vi "Dashboard Main.vi"() -> ()   [LabVIEW 2020]
uses:
  52f2dcef-b32f-41dc-9262-467f65fbdc6c.vi
  <vilib>/Rock Robotics/Network Tables/NT Write String Array.vi
  <vilib>/Rock Robotics/Network Tables/NT Write Boolean.vi
  <vilib>/Rock Robotics/WPI/Dashboard/WPI_DashboardLogging Global.vi
panel:
  out "NT Connection":bool
  in  "Camera Settings Right":T1={"Frame Rate"=30, "Compression"=30, "Size"=1, "DB Camera Config"=FALSE} {"Frame Rate" scale=1.0..30.0; "Compression" scale=100.0..-1.0; "Size" items=["640x480", "320x240", "160x120"]}
  in  "Camera Name Right":string(combo)="No Camera Selection"
  out "Camera Perf":string
  in  "TCP":refnum<k5>
  in  "Rec Mode":enum32{"Stop", "Record", "Playback"}(radio)
  out "Robot IP":string
  out "Image Message":string="Timeout in Camera Communications"
  in  "Dashboard Tab":T2(tab)
  in  "Balance in Manual?":bool=TRUE
  in  "Preload Cone?":bool=TRUE
  out "IMU Roll":dbl
  out "IMU Pitch":dbl
  in  "AE Speed":dbl=0.08
  in  "Config AE":bool=TRUE
  in  "Reset Wrist":bool
  in  "Reset Cascade":bool
  out "Wrist":dbl=15.0
  out "Cascade":dbl=0.1
  in  "Auto Calibrate":bool=TRUE
  in  "Robot Selector":u16(ring) items=["2468", "2687"]
  in  "Manual Paths":string[](array[string])
  in  "Max Rotation":dbl=270.0
  in  "Max Translation":dbl=16.0
  in  "Deadband":dbl=0.1
  in  "Auto Selector":T3(ring)
  out "IMU":dbl(knob) scale=-180.0..180.0
  in  "Select Auto":string(combo)="Select Autonomous ..."
  out "Mode":T4(ring)=enum."Auto Disabled"
  out "Right Camera Perf":cluster{"Bandwidth (Mbps)":dbl, "FPS":dbl}
  out "Auto Picture":picture
  out "Cone":bool
  out "Cube":bool
  in  "Mid":bool=TRUE
  in  "High":bool=TRUE
  in  "Field Centric":bool
  out "Camera Image Right":T5(plugin-control)
  out "Tree":string(tree)
  # "HW"
  # "IMU"
  # "SWERVE"
  # "PATH VISUAL"
  # "MANIPULATOR"
  # "CONFIGURATION"
  # "FIELD CENTRIC"
  # "HIGH"
  # "MID"
  # "CUBE"
  # "CONE"
  # "BRUSHLESS"
  # "12V MISSING"
  # "SENSOR FAULT"
  # "BRAKE"
  # "COAST"
  # "CAN FAULT"
  # "REVERSE"
  # "FORWARD"
  # "CORRUPT"
  # "UPDATING"
  # "RECOVERY"
  # "BRUSHED"
  # "BRAKE"
  # "COAST"
  # "https://cdn8.bigcommerce.com/s-t3eo8vwp22/product_images/uploaded_images/fault-no-12v.gif"
  # "PIGEON 2"
  # "DAMAGED HARDWARE"
  # "BOOTLOADER"
  # "CAN FAULT"
  # "ROBOT DISABLED"
  # "ROBOT ENABLED"
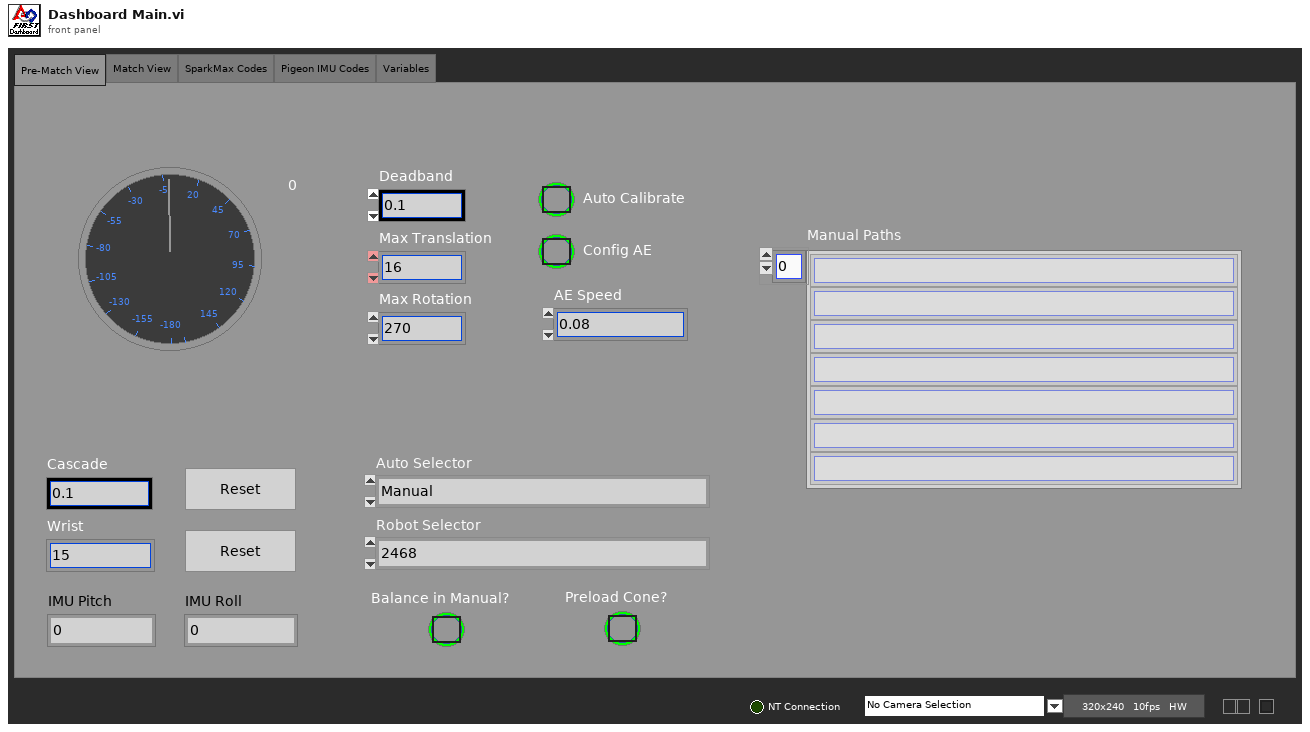
[diagram p1: front panel]
types:
  T1 = cluster{"Frame Rate":i32, "Compression":i32, "Size":u16, "DB Camera Config":bool}
  T2 = enum32{"Pre-Match View", "Match View", "SparkMax Codes", "Pigeon IMU Codes", "Variables"}
  T3 = enum16{"Manual", "FEEDER - 2.5 (2 High) + Balance", "FEEDER - 3 (2 High, 1 Low)", "WALL - 2 (High) + Balance", "WALL - 3 (2 High, 1 Low)", "MIDDLE - Wall Side 2 (High) + Balance", "MIDDLE - Feeder Side 2 (High) + Balance"}
  T4 = enum8{"Tele-Op Disabled", "Tele-Op Enabled", "Auto Disabled", "Auto Enabled", "Test Disabled", "Test Enabled", "Disconnected", "No Code", "E-Stop"}
  T5 = typedef "IMAQ Image.ctl" = refnum<image>
  T6 = cluster{"Save Path":path, "Interval (s)":dbl, "Keep":i32}
  T7 = typedef "Image Type" = u32
  T8 = cluster{"IDs":cluster{"RPC field ID":u16, "Unique ID":u16}, "String":string}
  T9 = cluster{"Dashboard Tab":refnum<vi>, "Rec Mode":refnum<vi>, "Tree":refnum<vi>, "Camera Perf":refnum<vi>, "Camera Settings Right":refnum<vi>, "Camera Name Right":refnum<vi>, "Camera Image Right":refnum<vi>}
  T10 = cluster{"Global Rectangle":i32[], "Contours":cluster{"Contour Type":u32, "ROI Type":u32, "Points":i32[]}[]}
  T11 = cluster{"Camera Name Right":string, string, "Saved DB Images Info":cluster{"Save Path":path, "Interval (s)":dbl, "Keep":i32}}
  T12 = cluster{"Error Strings":string, "Disable Counts":cluster{u16, u16}, "Rail Faults":cluster{u16, u16, u16}, "Robot IP":string, "DB Mode":u8, "Event Info":cluster{"Name":string, "Type":u8, "Number":u16, "Replay":u8}}
  T13 = cluster{"Storage":cluster{"Disk Free":u64, "RAM Block":u32, "RAM free":u32}, "CPU Utilization":cluster{"CPU % ISR":sgl, "CPU % Time Crit":sgl, "CPU % Timed Str":sgl, "CPU % High":sgl, "CPU % Above":sgl, "CPU % Normal":sgl, "CPU % Low":sgl}, "CAN":cluster{"% Bus Utilization":sgl, "Bus Off Cnt":u32, "TX_FIFO Full Cnt":u32, "Receive Error Cnt":u8, "Transmit Error Cnt":u8}, "HID":cluster{"HID Outputs":u32, "Rumble Low":u16, "Rumble High":u16}[]}
  T14 = cluster{"Status bits":cluster{"Test Mode":bool, "Autonomous":bool, "Enabled":bool, "Code Start":bool, "Brownout":bool, "Reserved 2":bool, "Reserved 3":bool, "E-Stop":bool}, "Code Trace":cluster{"Disabled":bool, "TeleOp":bool, "Auto":bool, "Test":bool}, "Controller Type":enum16{"unknown", "cRIO", "roboRio"}, "Code?":enum16{"unknown", "noCode", "code"}, "Battery V":dbl}
  T15 = cluster{"Control Bits":cluster{"TestMode":bool, "Autonomous":bool, "Enabled":bool, "FMS Present":bool, bool, bool, bool, "E-Stop":bool}, "Team Station ":u8, "Countdown":sgl, "Joystick Values":cluster{"Axes":dbl[], "Buttons":bool[], "POVs":i16[]}[]}
  T16 = typedef "imagedata.ctl" = cluster{"image type":i32, "image depth":i32, "image":u8[], "mask":u8[], "colors":u32[], "Rectangle":cluster{"left":i16, "top":i16, "right":i16, "bottom":i16}}
  T17 = cluster{"Operation":enum16{"Update", "Clear"}, "Color Box":u32}[]
  T18 = cluster{"Image Size":bool, "Image Type":bool, "Pixel Value":bool, "ROI Information":bool, "Zoom Factor":bool}
  T19 = cluster{"Shift":bool, "Ctrl":bool, "Alt":bool, "Cmd":bool, "Opt":bool}
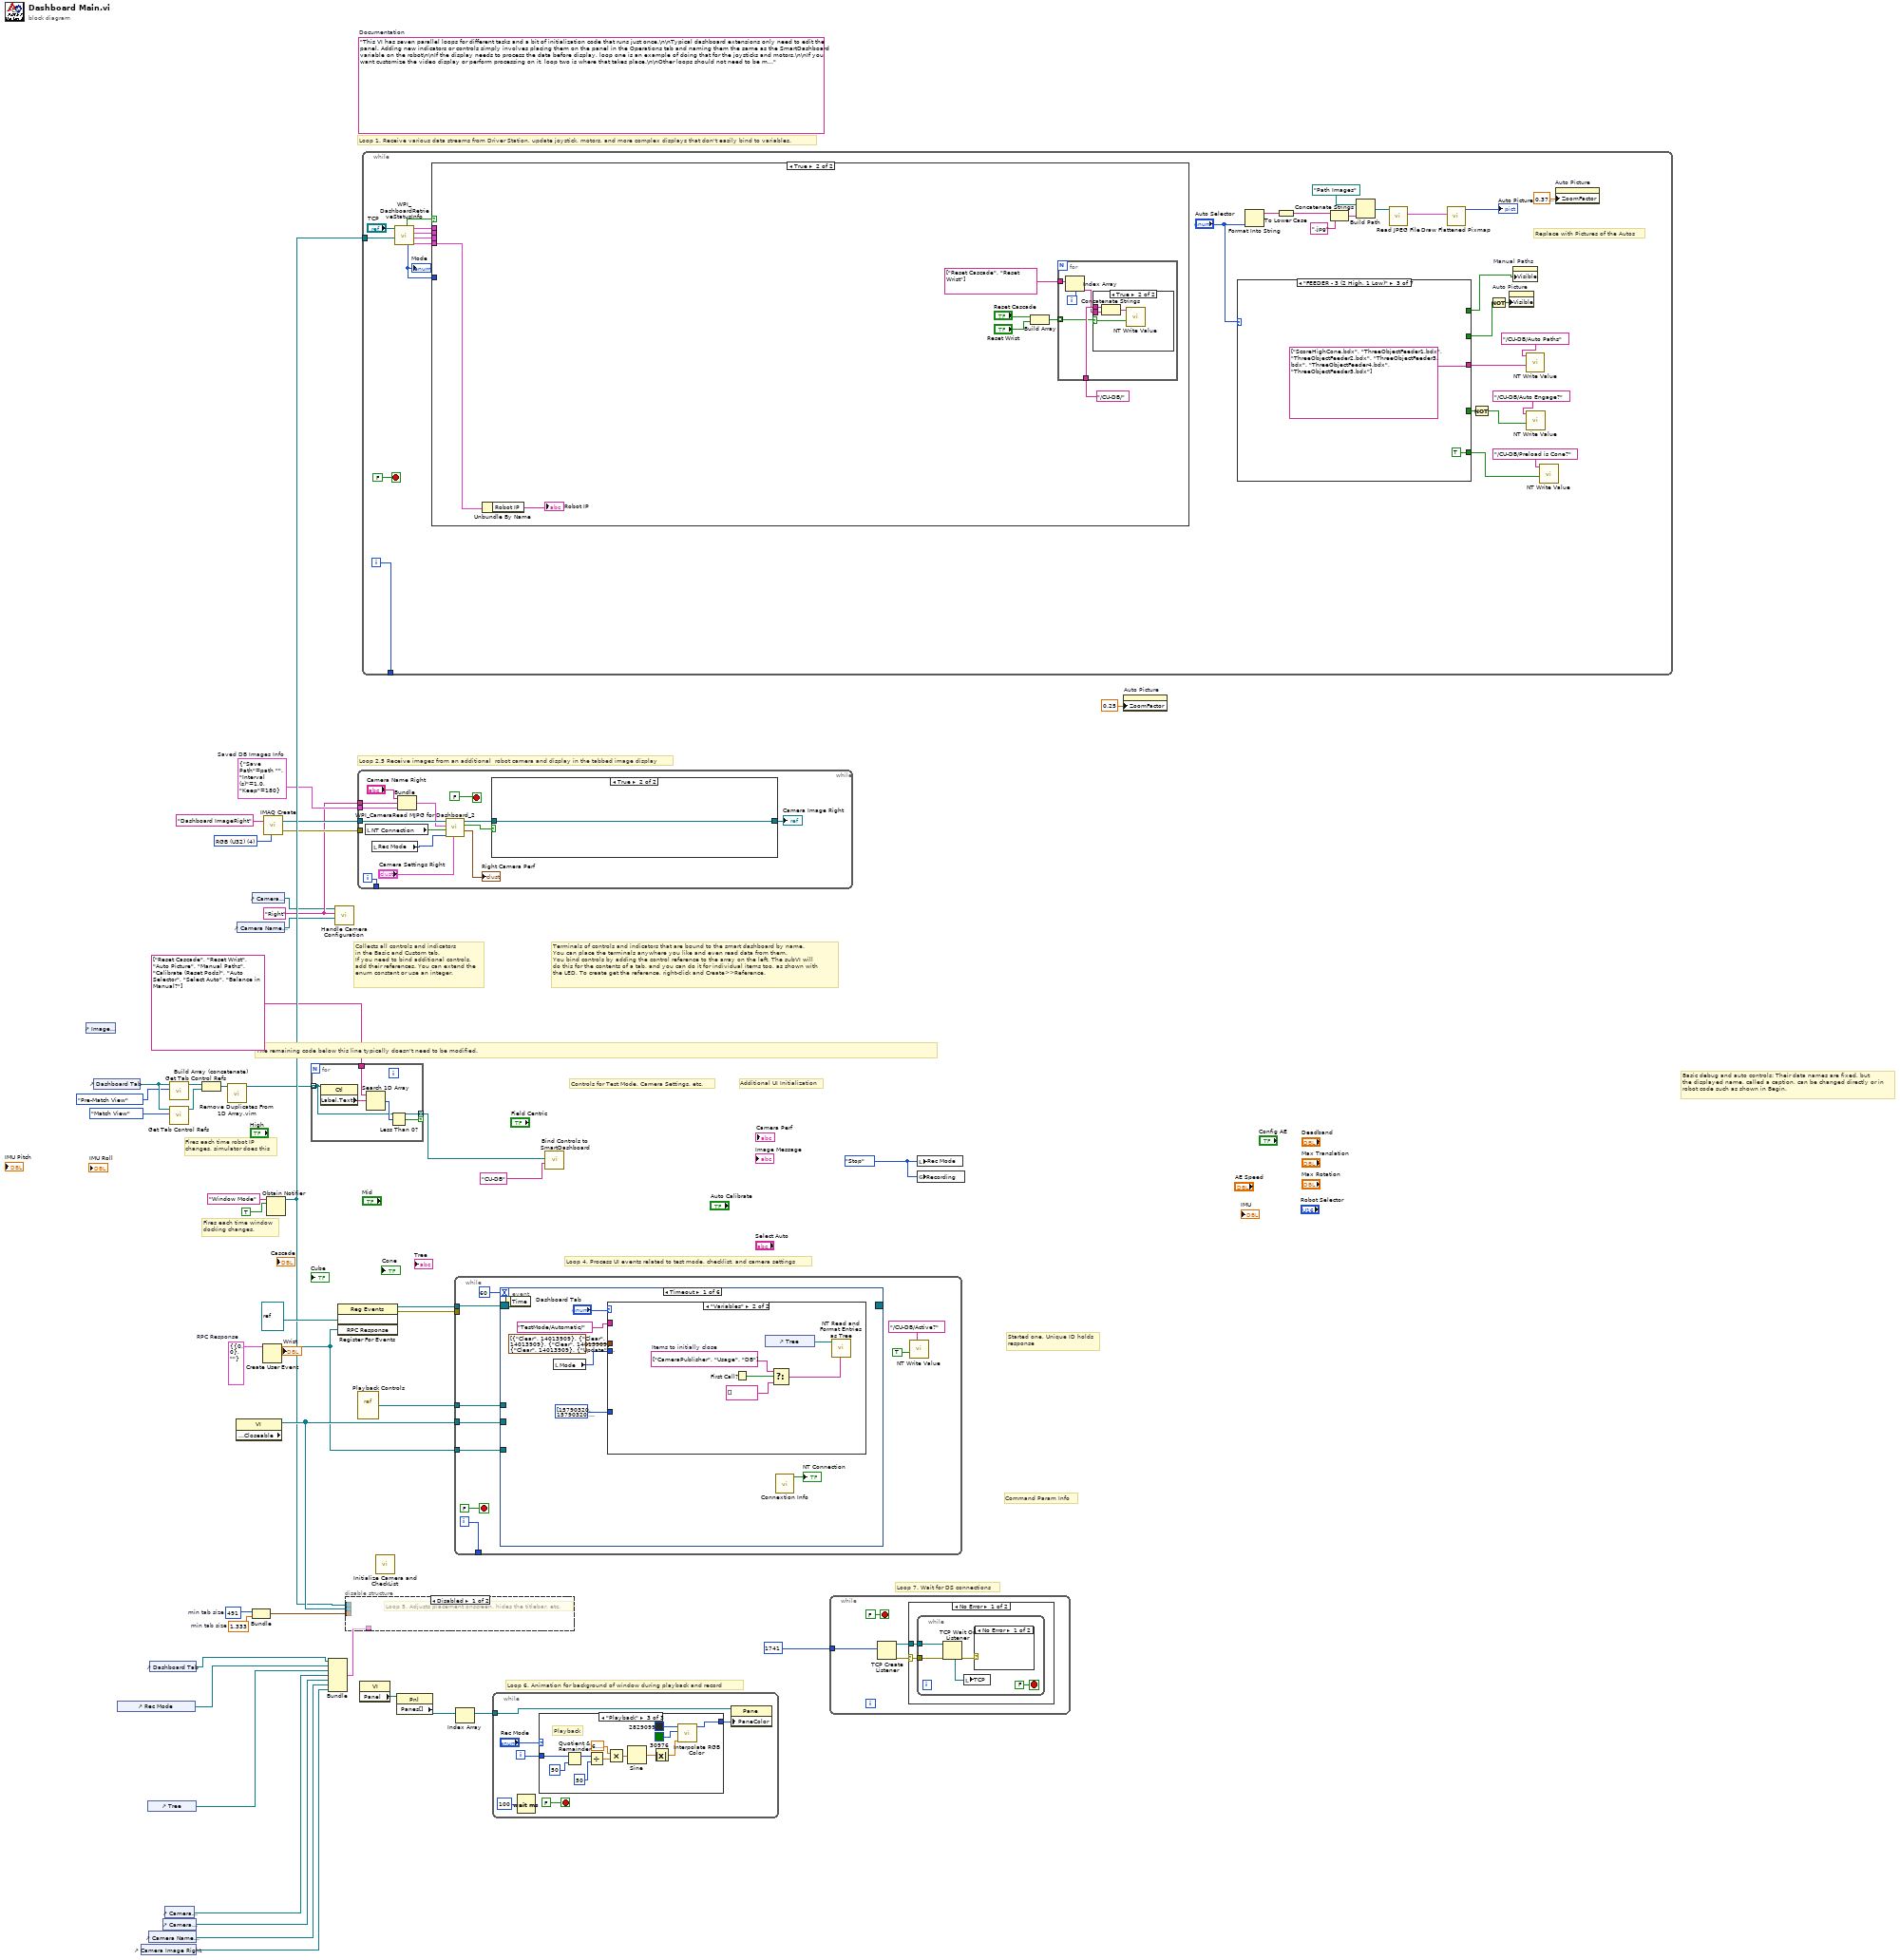
[diagram p0: block diagram]
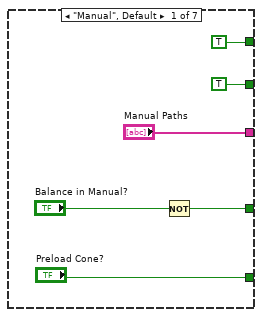
[diagram p2: hidden frame]
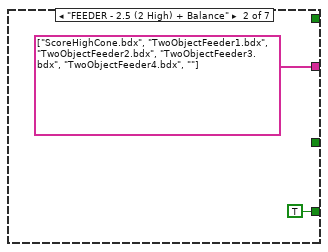
[diagram p3: hidden frame]
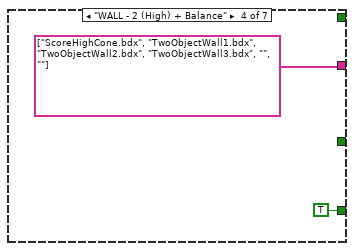
[diagram p4: hidden frame]
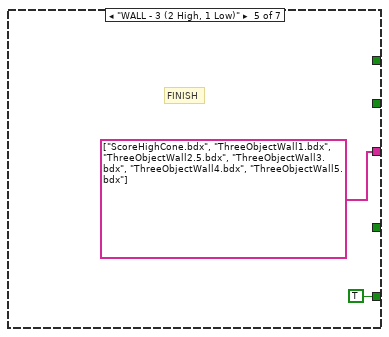
[diagram p5: hidden frame]
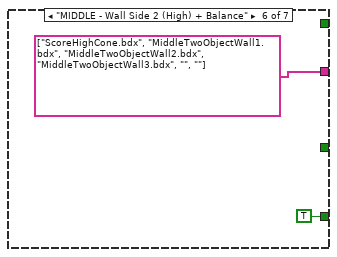
[diagram p6: hidden frame]
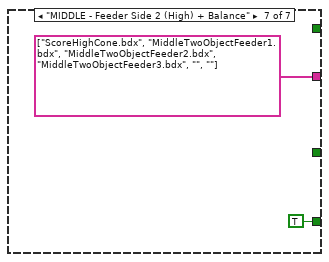
[diagram p7: hidden frame]
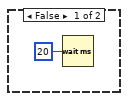
[diagram p8: hidden frame]
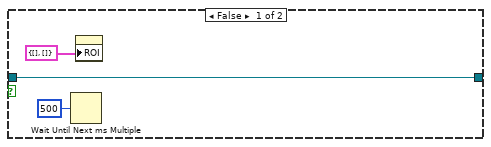
[diagram p11: hidden frame]
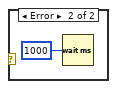
[diagram p12: hidden frame]
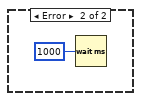
[diagram p13: hidden frame]
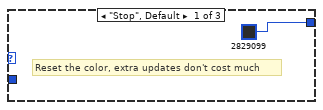
[diagram p14: hidden frame]
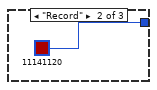
[diagram p15: hidden frame]
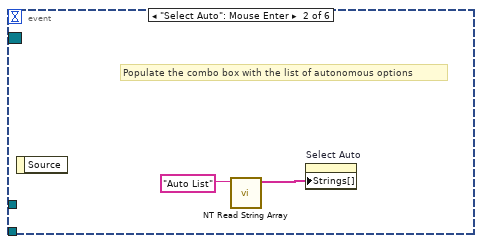
[diagram p17: hidden frame]
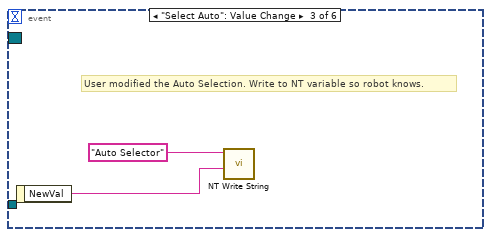
[diagram p18: hidden frame]
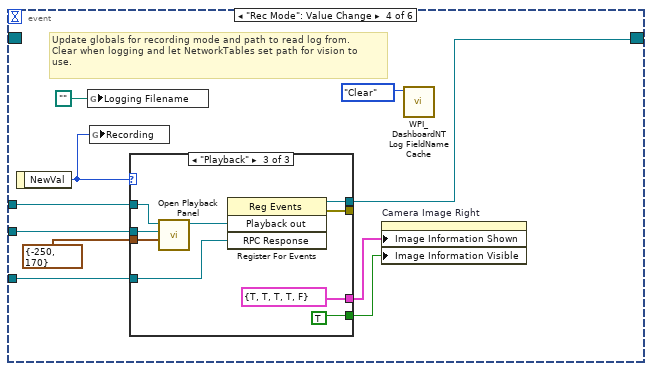
[diagram p19: hidden frame]
diagram:
  w17 = T6 {"Save Path"=path "", "Interval (s)"=1.0, "Keep"=180}  # Saved DB Images Info
  w16 = "Right"
  w23 = T7 4 items=["Grayscale (U8)", "Grayscale (I16)", "Grayscale (SGL)", "Complex (CSG)", "RGB (U32)", "HSL (U32)", "RGB (U64)"] ("Image Type")
  w27 = T8 {"IDs"={"RPC field ID"=0, "Unique ID"=0}, "String"=""}  # RPC Response
  w34 = 491  # min tab size
  w33 = 1.333  # min tab size
  w36 = enum32{"Stop", "Record", "Playback"}."Stop" ("Rec Mode")
  (unwired) "This VI has seven parallel loops for different tasks and a bit of initialization code that runs just once.\n\nTypical dashboard extensions only need to edit the panel. Adding new indicators or controls simply involves placing them on the panel in the Operations tab and naming them the same as the SmartDashboard variable on the robot\n\nIf the display needs to process the data before display, loop one is an example of doing that for the joysticks and motors.\n\nIf you want customize the video display or perform processing on it, loop two is where that takes place.\n\nOther loops should not need to be modified. They are pretty standard, and document the task they perform."  # Documentation
  # "Loop 2.5 Receive images from an additional  robot camera and display in the tabbed image display"
  # "Command Param Info"
  # "Started one, Unique ID holds\nresponse"
  # "Loop 7. Wait for DS connections"
  # "Basic debug and auto controls: Their data names are fixed, but\nthe displayed name, called a caption, can be changed directly or in\nrobot code such as shown in Begin."
  # "Controls for Test Mode, Camera Settings, etc."
  # "Additional UI Initialization"
  # "Loop 6. Animation for background of window during playback and record"
  # "Fires each time robot IP\nchanges, simulator does this"
  # "Fires each time window\ndocking changes."
  # "Collects all controls and indicators\nin the Basic and Custom tab.\nIf you need to bind additional controls,\nadd their references. You can extend the\nenum constant or use an integer."
  # "The remaining code below this line typically doesn't need to be modified."
  # "Loop 4. Process UI events related to test mode, checklist, and camera settings"
  # "Terminals of controls and indicators that are bound to the smart dashboard by name.\nYou can place the terminals anywhere you like and even read data from them.\nYou bind controls by adding the control reference to the array on the left. The subVI will\ndo this for the contents of a tab, and you can do it for individual items too, as shown with\nthe LED. To create get the reference, right-click and Create>>Reference."
  # "Loop 1. Receive various data streams from Driver Station, update joystick, motors, and more complex displays that don't easily bind to variables."
  n1 = control-ref of="Image Message"() -> ()  [unwired: 1 out]
  n2 = control-ref of="Dashboard Tab"() -> (w13:refnum<vi>)
  n3 = control-ref of="Rec Mode"() -> (w30:refnum<vi>)
  n4 = control-ref of="Camera Image Right"() -> (w18:refnum<vi>)
  n5 = control-ref of="Tree"() -> (w15:refnum<vi>)
  n6 = control-ref of="Camera Name Right"() -> (w19:refnum<vi>)
  n7 = control-ref of="Dashboard Tab"() -> (w5:refnum<vi>)
  n8 = control-ref of="Camera Settings Right"() -> (w20:refnum<vi>)
  n9 = control-ref of="Camera Perf"() -> (w25:refnum<vi>)
  n10 = call <vilib>:"Get Tab Control Refs.vi"("Page Index"=T2."Pre-Match View" ("Dashboard Tab"), "TabControl in"=w13) -> ("ControlsOnPage"=w12:refnum<vi>[])  [unwired: 9 in]
  n11 = call <vilib>:"Get Tab Control Refs.vi"("Page Index"=T2."Match View" ("Dashboard Tab"), "TabControl in"=w13) -> ("ControlsOnPage"=w11:refnum<vi>[])  [unwired: 9 in]
  n12 = Build Array (concatenate)(w12, w11) -> (w10:refnum<vi>[])
  n13 = call "Remove Duplicates From 1D Array.vim"("array"=w10) -> ("array with duplicates removed"=w7:refnum<vi>[])  [unwired: 10 in]
  n14 = property class="VI" props=["Front Panel.Closeable"]() -> (reference out=w35:refnum<vi>)  [unwired: 2 in, 2 out]
  n15 = control-ref of="Camera Name Right"() -> (w1:refnum<vi>)
  n16 = control-ref of="Camera Settings Right"() -> (w2:refnum<vi>)
  n17 = Bundle("min tab size"=w34, "min tab size"=w33) -> (w32:cluster{"min tab size":i32, "min tab size":dbl})  [unwired: 1 in]
  n18 = Create User Event(user event datatype=w27) -> (user event=w26:refnum<user-event>)  [unwired: 1 in, 1 out]
  n19 = call "IMAQ Create"("Image Name"="Dashboard ImageRight", "Image Type"=w23) -> ("New Image"=w22:T5, "error out"=w21:errorcluster)  [unwired: 2 in, 1 out]
  n20 = Obtain Notifier(name (unnamed)="Window Mode", notification data type=TRUE) -> (notifier out=w29:refnum<notifier>)  [unwired: 2 in, 2 out]
  n21 = for {
    tunnel: string[] ["Reset Cascade", "Reset Wrist", "Auto Picture", "Manual Paths", "Calibrate (Reset Pods)", "Auto Selector", "Select Auto", "Balance in Manual?"] -> [w50]
    tunnel: w7 -> [w47] mode=indexing
    tunnel: [w47] -> w6 mode=indexing if=w46
    n22 = property class="Ctl"(reference=w47) -> ("Label.Text"=w49:string)  [unwired: 1 in, 2 out]
    n23 = Search 1D Array(1D array=w50, element=w49) -> (index of element=w48:i32)  [unwired: 1 in]
    n24 = Less Than 0?(x=w48) -> (x < 0?=w46:bool)
  }
  n25 = Bundle("Dashboard Tab"=w5, "Rec Mode"=w30, "Tree"=w15, "Camera Perf"=w25, "Camera Settings Right"=w20, "Camera Name Right"=w19, "Camera Image Right"=w18) -> (w31:T9)  [unwired: 1 in]
  n26 = call "Handle Camera Configuration.vi"("CameraNameRef"=w1, "Display Name"=w16, "ClusterRef"=w2) -> ()  [unwired: 9 in]
  n27 = register-events(refnum<vi> refnum, w26) -> (reference out=w39:refnum<event-registration>, error out=w38:errorcluster)  [unwired: 2 in]
  n28 = disable-structure shown="Disabled" {
    disable-tunnel: w35 -> [_ _]
    disable-tunnel: w32 -> [_ _]
    disable-tunnel: w31 -> [_ _]
    disable-tunnel: w29 -> [_ _]
    frame Disabled {
      # "Loop 5. Adjusts placement onscreen, hides the titlebar, etc."
    }
    frame Enabled {
    }
  }
  n29 = while {
    tunnel: w22 -> [w64]
    tunnel: w21 -> [_]
    tunnel: [w59] -> _
    tunnel: w17 -> [w55]
    tunnel: w16 -> [w52]
    i -> [w59]
    stop <- FALSE stop-if-true
    n30 = local read "NT Connection"() -> (w56:bool)
    n31 = local read "Rec Mode"() -> (w63:enum32{"Stop", "Record", "Playback"})
    n32 = Bundle("Camera Name Right"="Camera Name Right", w52, "Saved DB Images Info"=w55) -> (w54:T11)  [unwired: 1 in]
    n33 = call <vilib>:"WPI_CameraRead MJPG for Dashboard_2.vi"("Camera Settings"="Camera Settings Right", "Rec Mode"=w63, "NT Connection"=w56, "Capture Info"=w54, "Image in"=w64) -> ("perf info"=→"Right Camera Perf":cluster{"Bandwidth (Mbps)":dbl, "fps":dbl}, "Active"=w58:bool, "Image\\ out"=w61:T5)  [unwired: 4 in]
    n34 = case shown="True" w58 {
      tunnel: w61 -> [w66 w68]
      tunnel: [w66 w68] -> w57
      frame False {
        n35 = Wait Until Next ms Multiple(millisecond multiple=u32 500) -> ()  [unwired: 1 out]
        n36 = property on="Camera Image Right" class="ImageControl"("ROI"=T10 {"Global Rectangle"=[], "Contours"=[]}) -> ()  [unwired: 2 in, 2 out]
      }
      frame True {
      }
    }
    "Camera Image Right" <- w57
  }
  n37 = vi-ref "Playback Controls.vi"() -> (w40:refnum<vi>)
  n38 = property class="VI"() -> ("Panel"=w42:refnum<vi>)  [unwired: 2 in, 2 out]
  n39 = while {
    tunnel: [w97] -> _
    tunnel: w29 -> [w89]
    i -> [w97]
    stop <- FALSE stop-if-true
    # "Replace with Pictures of the Autos"
    n40 = call <vilib>:"WPI_DashboardRetrieveStatusInfo.vi"("Window Mode Notifier"=w89, "TCP Cnx"="TCP") -> ("Power and Errors"=w92:T12, "Robot Metrics"=w95:T13, "Status Info"=w96:T14, "Control Info"=w93:T15, "Robot Mode"=w91:T4, "Process?"=w94:bool)  [unwired: 4 in]
    "Mode" <- w91
    n41 = case shown="True" w94 {
      tunnel: w96 -> [_ _]
      tunnel: w95 -> [_ _]
      tunnel: w93 -> [_ _]
      tunnel: w92 -> [_ w124]
      tunnel: w91 -> [_ _]
      frame False {
        n42 = Wait (ms)(milliseconds to wait=u32 20) -> ()  [unwired: 1 out]
      }
      frame True {
        n43 = Unbundle By Name(w124) -> ("Robot IP"=→"Robot IP":string)
        n44 = Build Array("Reset Cascade", "Reset Wrist") -> (w118:bool[])
        n45 = for {
          tunnel: "/CU-DB/" ("Name") -> [w129]
          tunnel: w118 -> [w125] mode=indexing
          tunnel: string[] ["Reset Cascade", "Reset Wrist"] -> [w127]
          i -> [w128]
          n46 = Index Array(array=w127, index=w128) -> (element=w126:string)
          n47 = case shown="True" w125 {
            selector: w125 -> [_ w130]
            tunnel: w129 -> [_ w132]
            tunnel: w126 -> [_ w131]
            frame False {
            }
            frame True {
              n48 = Concatenate Strings(w132, w131) -> (w133:string)
              n49 = call-poly <vilib>:"NT Write Value.vi"("value"=w130, "name"=w133) -> ()  [unwired: 9 in, 1 out]
            }
          }
        }
      }
    }
    n50 = case shown="\"FEEDER - 3 (2 High, 1 Low)\"" "Auto Selector" {
      tunnel: ["Manual Paths" string[] ["ScoreHighCone.bdx", "TwoObjectFeeder1.bdx", "TwoObjectFeeder2.bdx", "TwoObjectFeeder3.bdx", "TwoObjectFeeder4.bdx", ""] ("Manual Paths") string[] ["ScoreHighCone.bdx", "ThreeObjectFeeder1.bdx", "ThreeObjectFeeder2.bdx", "ThreeObjectFeeder3.bdx", "ThreeObjectFeeder4.bdx", "ThreeObjectFeeder5.bdx"] ("Manual Paths") string[] ["ScoreHighCone.bdx", "TwoObjectWall1.bdx", "TwoObjectWall2.bdx", "TwoObjectWall3.bdx", "", ""] ("Manual Paths") string[] ["ScoreHighCone.bdx", "ThreeObjectWall1.bdx", "ThreeObjectWall2.5.bdx", "ThreeObjectWall3.bdx", "ThreeObjectWall4.bdx", "ThreeObjectWall5.bdx"] ("Manual Paths") string[] ["ScoreHighCone.bdx", "MiddleTwoObjectWall1.bdx", "MiddleTwoObjectWall2.bdx", "MiddleTwoObjectWall3.bdx", "", ""] ("Manual Paths") string[] ["ScoreHighCone.bdx", "MiddleTwoObjectFeeder1.bdx", "MiddleTwoObjectFeeder2.bdx", "MiddleTwoObjectFeeder3.bdx", "", ""] ("Manual Paths")] -> w83
      tunnel: [TRUE ("Visible") _ _ _ _ _ _] -> w82
      tunnel: [TRUE ("Visible") _ _ _ _ _ _] -> w81
      tunnel: [w101 _ _ _ _ _ _] -> w86
      tunnel: ["Preload Cone?" TRUE ("Preload is Cone?") TRUE ("Preload is Cone?") TRUE ("Preload is Cone?") TRUE ("Preload is Cone?") TRUE ("Preload is Cone?") TRUE ("Preload is Cone?")] -> w88
      frame "Manual", Default {
        n51 = Not(x="Balance in Manual?") -> (.not. x?=w101:bool)
      }
      frame "FEEDER - 2.5 (2 High) + Balance" {
      }
      frame "FEEDER - 3 (2 High, 1 Low)" {
      }
      frame "WALL - 2 (High) + Balance" {
      }
      frame "WALL - 3 (2 High, 1 Low)" {
        # "FINISH"
      }
      frame "MIDDLE - Wall Side 2 (High) + Balance" {
      }
      frame "MIDDLE - Feeder Side 2 (High) + Balance" {
      }
    }
    n52 = Format Into String("Auto Selector") -> (resulting string=w75:string)  [unwired: 3 in, 1 out]
    n53 = To Lower Case(string=w75) -> (all lower case string=w76:string)
    n54 = Concatenate Strings(w76, ".jpg" ("string")) -> (w77:string)
    n55 = Build Path(base path=path "Path Images", name or relative path=w77) -> (appended path=w85:path)
    n56 = call <vilib>:"Read JPEG File.vi"("path to JPEG file"=w85) -> ("image data"=w84:T16)  [unwired: 8 in, 2 out]
    n57 = call <vilib>:"Draw Flattened Pixmap.vi"("image data"=w84) -> ("new picture"=→"Auto Picture":picture)  [unwired: 8 in]
    n58 = Not(x=w86) -> (.not. x?=w87:bool)
    n59 = Not(x=w82) -> (.not. x?=w79:bool)
    n60 = property on="Auto Picture" class="Pict"("Visible"=w79) -> ()  [unwired: 2 in, 2 out]
    n61 = property on="Manual Paths" class="Arr (strict)"("Visible"=w81) -> ()  [unwired: 2 in, 2 out]
    n62 = call-poly <vilib>:"NT Write Value.vi"("value"=w83, "name"="/CU-DB/Auto Paths") -> ()  [unwired: 9 in, 1 out]
    n63 = call-poly <vilib>:"NT Write Value.vi"("value"=w87, "name"="/CU-DB/Auto Engage?") -> ()  [unwired: 9 in, 1 out]
    n64 = call-poly <vilib>:"NT Write Value.vi"("value"=w88, "name"="/CU-DB/Preload is Cone?") -> ()  [unwired: 9 in, 1 out]
    n65 = property on="Auto Picture" class="Pict"("ZoomFactor"=sgl 0.38 ("Zoom Factor")) -> ()  [unwired: 2 in, 2 out]
  }
  n66 = call "Initialize Camera and CheckList.vi"() -> ()  [unwired: 12 in]
  n67 = property class="Pnl"(reference=w42) -> ("Panes[]"=w43:refnum<vi>[])  [unwired: 1 in, 2 out]
  n68 = while {
    tunnel: [w140] -> _
    tunnel: w40 -> [w139]
    tunnel: w39 -> [w138]
    tunnel: w38 -> [_]
    tunnel: w35 -> [w137]
    tunnel: w26 -> [w136]
    i -> [w140]
    stop <- FALSE stop-if-true
    n69 = event shown="[0] Timeout" {
      selector: w138 -> [_ _ _ _ _ _]
      dyn-events: [_ _ _ w164 _ _] -> _
      timeout: u32 60 ("milliseconds to wait") -> [_ _ _ _ _ _]
      tunnel: w139 -> [_ _ _ w166 w181 _]
      tunnel: w137 -> [_ _ _ w162 _ _]
      tunnel: w136 -> [_ _ _ w160 _ _]
      event Timeout {
        n70 = event-data() -> ()  [unwired: 1 in, 1 out]
        n71 = local read "Mode"() -> (w145:T4)
        n72 = case shown="\"Variables\"" "Dashboard Tab" {
          tunnel: "TestMode/Automatic/" ("Name Pattern") -> [_ _]
          tunnel: T17 [{"Operation"=enum."Clear", "Color Box"=14013909}, {"Operation"=enum."Clear", "Color Box"=14013909}, {"Operation"=enum."Clear", "Color Box"=14013909}, {"Operation"=enum."Clear", "Color Box"=14013909}, {"Operation"=enum."Update", "Color Box"=14013909}, {"Operation"=enum."Update", "Color Box"=16777215}, {"Operation"=enum."Clear", "Color Box"=14013909}, {"Operation"=enum."Clear", "Color Box"=14013909}, {"Operation"=enum."Clear", "Color Box"=14013909}] -> [_ _]
          tunnel: w145 -> [_ _]
          tunnel: u32[] [15790320, 15790320, 15790320, 15790320, 16777215, 16777215, 15790320, 15790320, 15790320] -> [_ _]
          frame Default {
          }
          frame "Variables" {
            w151 = string[] ["CameraPublisher", "Usage", "DB"]  # Items to initially close
            n73 = First Call?() -> (First Call?: T/F=w152:bool)
            n74 = control-ref of="Tree"() -> (w153:refnum<vi>)
            n75 = Select(t=w151, s=w152, f=string[] []) -> (s? t:f=w149:string[])
            n76 = call <vilib>:"NT Read and Format Entries as Tree.vi"("Tags to  Close"=w149, "Tree Refnum"=w153) -> ()  [unwired: 8 in, 2 out]
          }
        }
        n77 = call <vilib>:"Connextion Info.vi"() -> ("Connected"=→"NT Connection":bool)  [unwired: 10 in, 1 out]
      }
      event "Select Auto": Mouse Enter {
        # "Populate the combo box with the list of autonomous options"
        n78 = event-data() -> ()  [unwired: 1 in, 1 out]
        n79 = call <vilib>:"NT Read String Array.vi"("name"="Auto List" ("Name")) -> ("value"=w154:string[])  [unwired: 8 in, 2 out]
        n80 = property on="Select Auto" class="CmbBox"("Strings[]"=w154) -> ()  [unwired: 2 in, 2 out]
      }
      event "Select Auto": Value Change {
        # "User modified the Auto Selection. Write to NT variable so robot knows."
        n81 = event-data() -> ("NewVal"=w156:string)  [unwired: 1 in]
        n82 = call <vilib>:"NT Write String.vi"("value"=w156, "name"="Auto Selector" ("Name")) -> ()  [unwired: 9 in, 1 out]
      }
      event "Rec Mode": Value Change {
        # "Update globals for recording mode and path to read log from.\nClear when logging and let NetworkTables set path for vision to\nuse."
        n83 = event-data() -> ("NewVal"=w167:enum32{"Stop", "Record", "Playback"})  [unwired: 1 in]
        n84 = global write "WPI_DashboardLogging Global.vi" "Logging Filename"(path "") -> ()
        n85 = global write "WPI_DashboardLogging Global.vi" "Recording"(w167) -> ()
        n86 = case shown="\"Playback\"" w167 {
          tunnel: w166 -> [_ w169 w178]
          tunnel: [_ _ w177] -> w164
          tunnel: [_ _ w176] -> _
          tunnel: w162 -> [_ _ w174]
          tunnel: cluster{i32, i32} {-250, 170} -> [_ _ w173]
          tunnel: [_ _ T18 {"Image Size"=TRUE, "Image Type"=TRUE, "Pixel Value"=TRUE, "ROI Information"=TRUE, "Zoom Factor"=FALSE} ("Image Information Shown:All Elements")] -> w158
          tunnel: [_ _ TRUE ("Zoom Factor")] -> w159
          tunnel: w160 -> [_ _ w170]
          frame Default {
          }
          frame "Stop", "Record" {
            # "Place Window too"
            n87 = invoke class="VI" method="FP.Close"(reference=w169) -> (reference out=w168:refnum<vi>)  [unwired: 2 in, 2 out]
            n88 = invoke class="VI" method="Abort VI"(reference=w168) -> ()  [unwired: 2 in, 3 out]
          }
          frame "Playback" {
            n89 = call "Open Playback Panel.vi"("Offset"=w173, "DB VI Ref"=w174, "Playback in"=w178) -> ("Playback out"=w175:refnum<vi>)  [unwired: 8 in]
            n90 = register-events(w175, w170) -> (reference out=w177:refnum<event-registration>, error out=w176:errorcluster)  [unwired: 2 in]
          }
        }
        n91 = property on="Camera Image Right" class="ImageControl"("Image Information Shown"=w158, "Image Information Visible"=w159) -> ()  [unwired: 2 in, 2 out]
        n92 = call <vilib>:"WPI_DashboardNT Log FieldName Cache.vi"("Operation"=enum16{"Lookup/Add", "Index", "Clear"}."Clear") -> ()  [unwired: 8 in, 3 out]
      }
      event Panel Close {
        # "Abort playback window and ourself"
        n93 = event-data() -> ()  [unwired: 1 in, 4 out]
        n94 = invoke class="VI" method="FP.Close"(reference=w181) -> (reference out=w180:refnum<vi>)  [unwired: 2 in, 2 out]
        n95 = invoke class="VI" method="Abort VI"(reference=w180) -> (error out=w179:errorcluster)  [unwired: 2 in, 2 out]
        n96 = invoke class="VI" method="Abort VI"(error in=w179) -> ()  [unwired: 2 in, 3 out]
      }
      event "Tree": Double Click {
        n97 = event-data() -> ("PlatMods"=w187:T19, "Tag"=w184:string)  [unwired: 1 in]
        n98 = Unbundle(w187) -> ("Shift"=w186:bool)  [unwired: 4 out]
        n99 = String Subset(string=w184, length (rest)=1 ("length (rest)")) -> (substring=w183:string)  [unwired: 1 in]
        n100 = Not(x=w186) -> (.not. x?=w185:bool)
        n101 = case shown="\"/\"" w183 {
          tunnel: w184 -> [_ w189]
          tunnel: w185 -> [_ w188]
          frame Default {
          }
          frame "/" {
            n102 = call <vilib>:"NT Update Persistence.vi"("Persistence"=w188, "Name"=w189) -> ()  [unwired: 9 in, 1 out]
          }
        }
      }
    }
    n103 = call-poly <vilib>:"NT Write Value.vi"("value"=TRUE ("Boolean"), "name"="/CU-DB/Active?" ("Name")) -> ()  [unwired: 9 in, 1 out]
  }
  n104 = Index Array(array=w43) -> (element=w41:refnum<vi>)  [unwired: 1 in]
  n105 = while {
    tunnel: w41 -> [w191]
    i -> [w194]
    stop <- FALSE stop-if-true
    n106 = Wait (ms)(milliseconds to wait=u32 100) -> ()  [unwired: 1 out]
    n107 = case shown="\"Playback\"" "Rec Mode" {
      tunnel: w194 -> [_ _ w209]
      tunnel: [u32 2829099 ("Base Color") u32 11141120 ("Target Color") w198] -> w190
      frame "Stop", Default {
        # "Reset the color, extra updates don't cost much"
      }
      frame "Record" {
      }
      frame "Playback" {
        # "Playback"
        n108 = Quotient & Remainder(x=w209, y=u32 50 ("milliseconds to wait")) -> (x-y*floor(x/y)=w205:u32)  [unwired: 1 out]
        n109 = Divide(x=w205, y=u32 50 ("milliseconds to wait")) -> (x/y=w202:dbl)
        n110 = Multiply(x=6.283185307179586, y=w202) -> (x*y=w207:dbl)
        n111 = Sine(x=w207) -> (sin(x)=w206:dbl)
        n112 = Absolute Value(x=w206) -> (abs(x)=w199:dbl)
        n113 = call "Interpolate RGB Color.vi"("Proportion"=w199, "Target Color"=u32 30976, "Base Color"=u32 2829099) -> ("Result Color"=w198:u32)  [unwired: 8 in]
      }
    }
    n114 = property class="Pane"(reference=w191, "PaneColor"=w190) -> ()  [unwired: 1 in, 2 out]
  }
  n115 = call <vilib>:"Bind Controls to SmartDashboard.vi"("Path Prefix"="CU-DB", "Bound Control Refs"=w6) -> ()  [unwired: 10 in]
  n116 = while {
    tunnel: u16 1741 ("timeout ms (25000)") -> [w211]
    stop <- FALSE stop-if-true
    n117 = TCP Create Listener(10:w211) -> (0:w210:errorcluster, 3:w212:refnum<k5>)  [unwired: 4 in, 1 out]
    n118 = case shown="No Error" w210 {
      selector: w210 -> [w214 _]
      tunnel: w212 -> [w215 _]
      frame No Error {
        n119 = while {
          tunnel: w215 -> [w218]
          tunnel: w214 -> [w217]
          stop <- FALSE stop-if-true
          n120 = TCP Wait On Listener(8:w217, 11:w218) -> (0:w219:errorcluster, 4:w220:refnum<k5>)  [unwired: 2 in, 3 out]
          n121 = local write "TCP"(w220) -> ()
          n122 = case shown="No Error" w219 {
            frame No Error {
            }
            frame Error {
              n123 = Wait (ms)(milliseconds to wait=u32 1000) -> ()  [unwired: 1 out]
            }
          }
        }
      }
      frame Error {
        n124 = Wait (ms)(milliseconds to wait=u32 1000) -> ()  [unwired: 1 out]
      }
    }
  }
  n125 = global write "WPI_DashboardLogging Global.vi" "Recording"(w36) -> ()
  n126 = local write "Rec Mode"(w36) -> ()
  n127 = property on="Auto Picture" class="Pict"("ZoomFactor"=sgl 0.25 ("Zoom Factor")) -> ()  [unwired: 2 in, 2 out]
